vi "Update UI.vi"(7 "Target PCL Period":u32=10000 caption="Target Period" format="%d us", 8 "error in (no error)":errorcluster, 10 "stop":bool, 11 "UI Pointers":T1) -> (0 "error out":errorcluster, 1 "Framework Iteration":i32 format="%d cycles", 2 "stop?":bool, 3 "Actual Frequency":dbl format="%.1pHz", 5 "Actual Period":u32 format="%d us")   [LabVIEW 2017]
uses:
  User Interface Pointers.ctl
  <vilib>/NI/Memory Manager/Classes/Pointer/Pointer.lvclass
  <vilib>/NI/Memory Manager/Classes/Pointer/Pointer.lvclass/Pointer.ctl
  <vilib>/NI/Memory Manager/Classes/Pointer/Write Bool.vi
  <vilib>/NI/Memory Manager/Classes/Pointer/Read Bool.vi
  <vilib>/NI/Memory Manager/Classes/Pointer/Read U32.vi
  <vilib>/NI/Memory Manager/Classes/Pointer/Write U32.vi
  <vilib>/NI/Memory Manager/Classes/Pointer/Read I32.vi
  <vilib>/NI/Memory Manager/Classes/Pointer/Write (No Check).vi
  <vilib>/NI/Memory Manager/Classes/Pointer/Write (No Check) Bool.vi
  <vilib>/NI/Memory Manager/Classes/Pointer/Check Move.vi
  <vilib>/NI/Memory Manager/Classes/Pointer/Read (No Check).vi
  <vilib>/NI/Memory Manager/Classes/Pointer/Read (No Check) Bool.vi
  <vilib>/NI/Memory Manager/Classes/Pointer/Read (No Check) U32.vi
  <vilib>/NI/Memory Manager/Classes/Pointer/Write (No Check) U32.vi
  <vilib>/NI/Memory Manager/Classes/Pointer/Read (No Check) I32.vi
  <vilib>/NI/Memory Manager/Classes/Pointer/Get Address.vi
  <vilib>/NI/Memory Manager/Classes/Pointer/Check Null Pointer.vi
  <vilib>/NI/Memory Manager/Classes/Pointer/Check Count.vi
  <vilib>/NI/Memory Manager/Classes/Pointer/Check Bounds (Power of 2).vi
  <vilib>/NI/Memory Manager/Classes/Pointer/Errors.vi
  <vilib>/NI/Memory Manager/Classes/Pointer/Null Pointer.vi
  <vilib>/NI/Memory Manager/Classes/Pointer/Is Null.vi
  <vilib>/NI/Memory Manager/Classes/Pointer/Get Size.vi
  <vilib>/NI/Memory Manager/Classes/Pointer/Out of Bounds.vi
  <vilib>/NI/Memory Manager/Classes/Pointer/Check Bounds.vi
  <vilib>/NI/Memory Manager/Classes/Pointer/Create Error.vi
  <vilib>/NI/Memory Manager/VIs/Source.Write.String.vi
  <vilib>/NI/Memory Manager/Classes/Pointer/Write Pointer Size.vi
  <vilib>/NI/Memory Manager/VIs/Source.Write.Scalar.Base10.vi
  <vilib>/NI/Memory Manager/VIs/Source.Write.Scalar.Base10 (U64).vi
  <vilib>/NI/Memory Manager/Classes/Pointer/Check Pointer Bounds.vi
  <vilib>/NI/Memory Manager/Classes/Pointer/Check Buffer Bounds.vi
  <vilib>/NI/Memory Manager/VIs/New Error Cluster Constant.vi
  <vilib>/NI/Memory Manager/VIs/New Error Cluster Constant (512B).vi
  <vilib>/NI/Memory Manager/VIs/Error Cluster.Set Status.vi
  <vilib>/NI/Memory Manager/VIs/Error Cluster.Set Code.vi
  <vilib>/NI/Memory Manager/VIs/Error Cluster.Set VI Source.vi
  <vilib>/NI/Memory Manager/Constants/Constants.vi
  <vilib>/NI/Memory Manager/Constants/Library Name.vi
  <vilib>/NI/Memory Manager/Classes/Pointer/Pointer Error Info.vi
  <vilib>/NI/Memory Manager/Constants/Pointer Class Name.vi
  <vilib>/NI/Memory Manager/Classes/Pointer/Buffer Underflow.vi
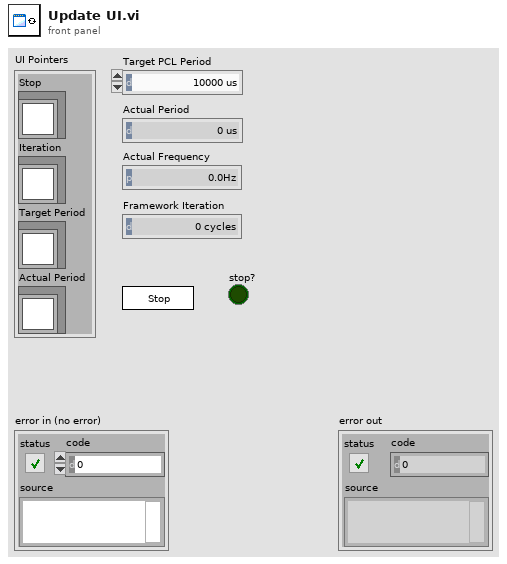
[diagram p1: front panel]
types:
  T1 = typedef "User Interface Pointers.ctl" = cluster{"Stop":refnum<class "Pointer.lvclass">, "Iteration":refnum<class "Pointer.lvclass">, "Target Period":refnum<class "Pointer.lvclass">, "Actual Period":refnum<class "Pointer.lvclass">}
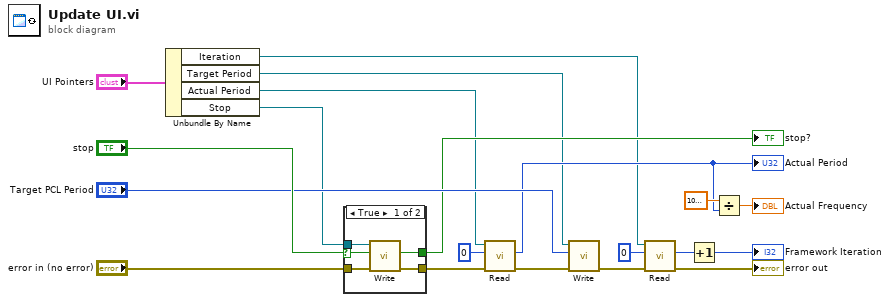
[diagram p0: block diagram]
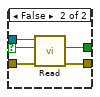
[diagram p2: hidden frame]
diagram:
  n1 = Unbundle By Name("UI Pointers") -> ("Iteration"=w3:refnum<class "Pointer.lvclass">, "Target Period"=w1:refnum<class "Pointer.lvclass">, "Actual Period"=w2:refnum<class "Pointer.lvclass">, "Stop"=w4:refnum<class "Pointer.lvclass">)
  n2 = case shown="True" "stop" {
    selector: "stop" -> [w23 w28]
    tunnel: [w25 w30] -> w11
    tunnel: w4 -> [w24 w29]
    tunnel: [w21 w27] -> w10
    tunnel: "error in (no error)" -> [w22 w26]
    frame True {
      n3 = call-poly <vilib>:"Write.vi"("error in (no error)"=w22, "buffer in"=w23, "Pointer in"=w24) -> ("error out"=w21:errorcluster, "buffer in"=w25:bool)  [unwired: 5 in, 2 out]
    }
    frame False {
      n4 = call-poly <vilib>:"Read.vi"("error in (no error)"=w26, "buffer in"=w28, "Pointer in"=w29) -> ("error out"=w27:errorcluster, "buffer out"=w30:bool)  [unwired: 5 in, 2 out]
    }
  }
  "stop?" <- w11
  n5 = call-poly <vilib>:"Read.vi"("error in (no error)"=w10, "buffer in"=u32 0, "Pointer in"=w2) -> ("error out"=w9:errorcluster, "buffer out"=w5:u32)  [unwired: 5 in, 2 out]
  "Actual Period" <- w5
  n6 = call-poly <vilib>:"Write.vi"("error in (no error)"=w9, "buffer in"="Target PCL Period", "Pointer in"=w1) -> ("error out"=w7:errorcluster)  [unwired: 5 in, 3 out]
  n7 = call-poly <vilib>:"Read.vi"("error in (no error)"=w7, "buffer in"=0, "Pointer in"=w3) -> ("error out"=→"error out":errorcluster, "buffer out"=w14:i32)  [unwired: 5 in, 2 out]
  n8 = Increment(x=w14) -> (x+1=→"Framework Iteration":i32)
  n9 = Divide(x=1000000.0, y=w5) -> (x/y=→"Actual Frequency":dbl)
